vi "Set Legends.vi"(8 "error in (no error)":errorcluster, 11 "[V] Waveform in":refnum<class "[V] Waveform.lvclass">) -> (0 "error out":errorcluster, 3 "[V] Waveform out":refnum<class "[V] Waveform.lvclass">)   [LabVIEW 2020, in "[V] Waveform.lvlib" / "[V] Waveform.lvclass"]
uses:
  [V] Waveform.lvclass
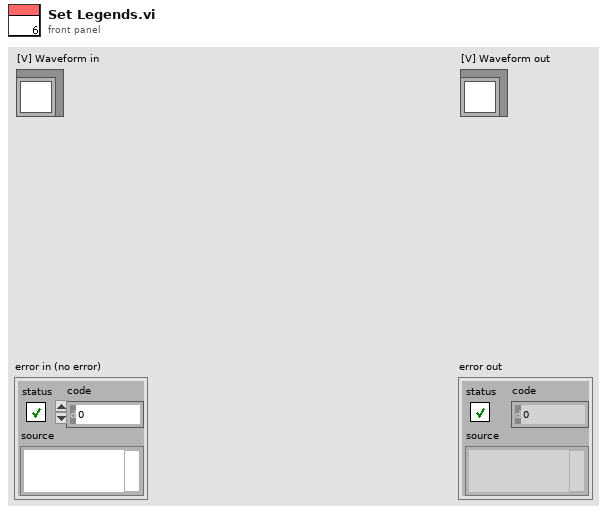
[diagram p1: front panel]
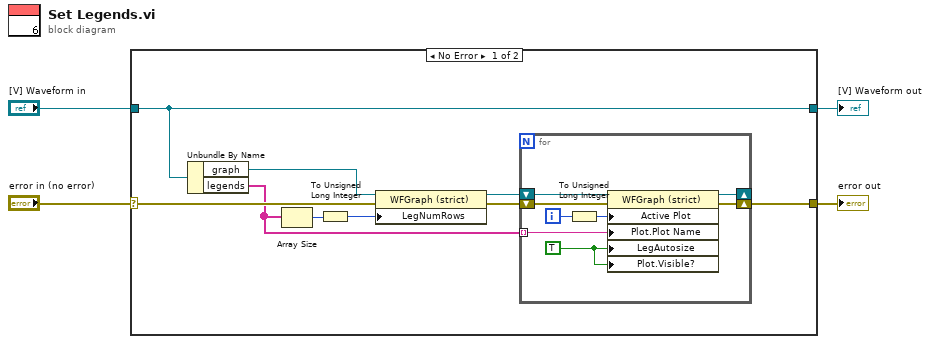
[diagram p0: block diagram]
diagram:
  n1 = case shown="No Error" "error in (no error)" {
    selector: "error in (no error)" -> [w12 w23]
    tunnel: [w6 w23] -> w3
    tunnel: [w13 w22] -> w1
    tunnel: "[V] Waveform in" -> [w13 w22]
    frame No Error {
      n2 = Unbundle By Name(w13) -> ("graph"=w11:refnum<vi>, "legends"=w5:string[])
      n3 = Array Size(array=w5) -> (size(s)=w10:i32)
      n4 = To Unsigned Long Integer(number=w10) -> (unsigned 32bit integer=w9:u32)
      n5 = property class="WFGraph (strict)"(reference=w11, error in=w12, "LegNumRows"=w9) -> (reference out=w7:refnum<vi>, error out=w8:errorcluster)
      n6 = for {
        shift-right: [w19] -> w6
        shift-left: w8 -> [w21]
        shift-right: [w18] -> _
        shift-left: w7 -> [w20]
        tunnel: w5 -> [w15] mode=indexing
        i -> [w17]
        w14 = TRUE ("Legend:Autosize")
        n7 = To Unsigned Long Integer(number=w17) -> (unsigned 32bit integer=w16:u32)
        n8 = property class="WFGraph (strict)"(reference=w20, error in=w21, "Active Plot"=w16, "Plot.Plot Name"=w15, "LegAutosize"=w14, "Plot.Visible?"=w14) -> (reference out=w18:refnum<vi>, error out=w19:errorcluster)
      }
    }
    frame Error {
    }
  }
  "error out" <- w3
  "[V] Waveform out" <- w1
